vi "Help Seal.vi"(0 "Signals":T2, 5 "Pressure Controls":T1, 7 "Seal Parameters":refnum<vi>, 9 "Suction Parameters":refnum<vi>, 11 "error in (no error)":errorcluster, 13 "Dialog Indicator":refnum<vi>, 14 "Abort":refnum<vi>) -> (10 "Seal":bool, 15 "error out":errorcluster)   [LabVIEW 2012, in "Autopatcher Daemon.lvlib"]
uses:
  Autopatcher Daemon.lvlib
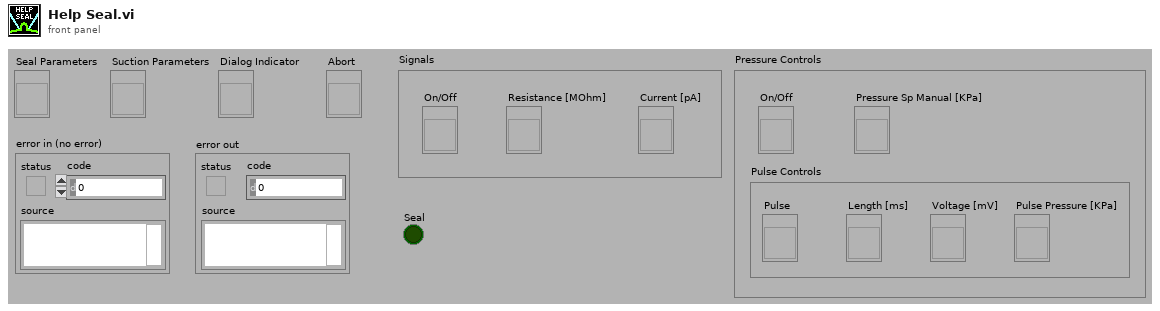
[diagram p1: front panel]
types:
  T1 = cluster{"On/Off":refnum<vi>, "Pulse Controls":cluster{"Pulse":refnum<vi>, "Length [ms]":refnum<vi>, "Voltage [mV]":refnum<vi>, "Pulse Pressure [KPa]":refnum<vi>}, "Pressure Sp Manual [KPa]":refnum<vi>}
  T2 = cluster{"On/Off":refnum<vi>, "Resistance [MOhm]":refnum<vi>, "Current [pA]":refnum<vi>}
  T3 = cluster{"Seal Target [MOhm]":dbl, "Stability Threhsold [%]":dbl, "Seal Timeout [s]":dbl, "Stability Refresh [ms]":dbl}
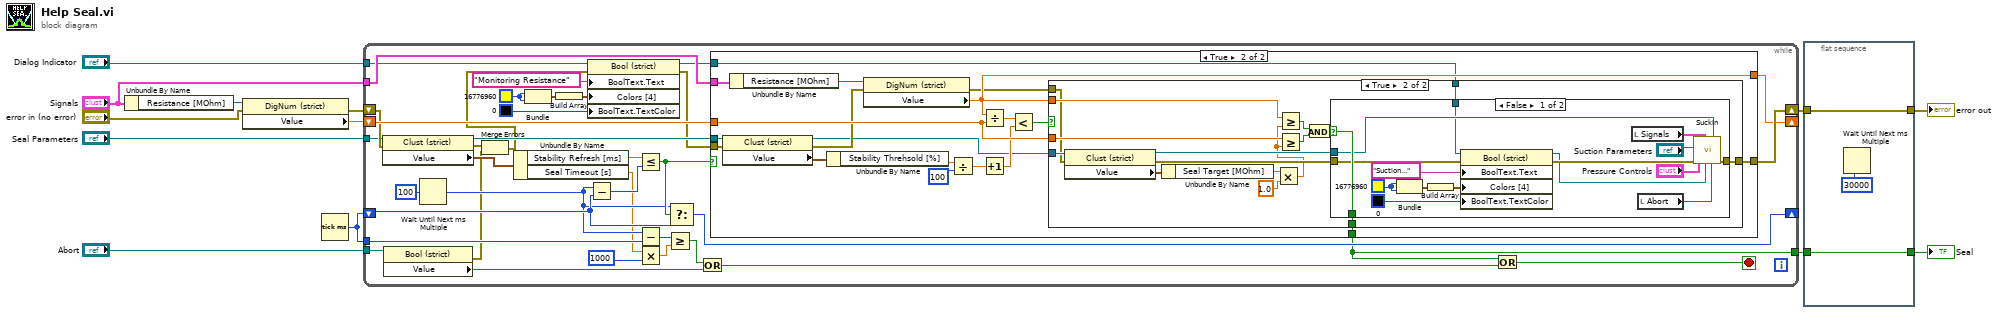
[diagram p0: block diagram]
diagram:
  n1 = Unbundle By Name("Signals") -> ("Resistance [MOhm]"=w12:refnum<vi>)
  n2 = property class="DigNum (strict)"(reference=w12, error in="error in (no error)") -> (error out=w10:errorcluster, "Value"=w11:dbl)  [unwired: 1 out]
  n3 = Tick Count (ms)() -> (millisecond timer value=w8:u32)
  n4 = while {
    shift-right: [w31] -> _
    shift-left: w8 -> [w50]
    tunnel: w8 -> [w47]
    shift-right: [w30] -> _
    shift-left: w11 -> [w45]
    tunnel: [w14] -> w13
    tunnel: "Abort" -> [w29]
    tunnel: "Signals" -> [w20]
    tunnel: "Seal Parameters" -> [w37]
    shift-right: [w43] -> w3
    shift-left: w10 -> [w38]
    tunnel: "Dialog Indicator" -> [w16]
    stop <- w44 stop-if-true
    w21 = u32 16776960
    n5 = property class="Clust (strict)"(reference=w37, error in=w38) -> (reference out=w36:refnum<vi>, error out=w27:errorcluster, "Value"=w35:T3)
    n6 = property class="Bool (strict)"(reference=w29) -> (error out=w26:errorcluster, "Value"=w33:bool)  [unwired: 1 in, 1 out]
    n7 = Wait Until Next ms Multiple(millisecond multiple=u32 100) -> (millisecond timer value=w39:u32)
    n8 = Merge Errors(w27, w26) -> (w18:errorcluster)
    n9 = Unbundle By Name(w35) -> ("Stability Refresh [ms]"=w15:dbl, "Seal Timeout [s]"=w28:dbl)
    n10 = Bundle(w21, w21) -> (w22:cluster{u32, u32})  [unwired: 1 in]
    n11 = Build Array(w22) -> (w23:cluster{u32, u32}[])
    n12 = property class="Bool (strict)"(reference=w16, error in=w18, "BoolText.Text"="Monitoring Resistance" ("Boolean Text.Text"), "Colors [4]"=w23, "BoolText.TextColor"=u32 0) -> (reference out=w17:refnum<vi>, error out=w19:errorcluster)
    n13 = Subtract(x=w39, y=w50) -> (x-y=w48:u32)
    n14 = Less Or Equal?(x=w15, y=w48) -> (x <= y?=w49:bool)
    n15 = Subtract(x=w39, y=w47) -> (x-y=w46:u32)
    n16 = Multiply(x=w28, y=u32 1000) -> (x*y=w40:dbl)
    n17 = Greater Or Equal?(x=w46, y=w40) -> (x >= y?=w34:bool)
    n18 = Select(t=w39, s=w49, f=w50) -> (s? t:f=w31:u32)
    n19 = Or(x=w34, y=w33) -> (x .or. y?=w41:bool)
    n20 = case shown="True" w49 {
      selector: w49 -> [w52 _]
      tunnel: w45 -> [w53 w70]
      tunnel: [w53 w67] -> w30
      tunnel: [w52 w69] -> w14
      tunnel: [w51 w68] -> w43
      tunnel: w20 -> [_ w55]
      tunnel: w36 -> [_ w60]
      tunnel: w19 -> [w51 w59]
      tunnel: w17 -> [_ w54]
      frame False {
      }
      frame True {
        n21 = property class="Clust (strict)"(reference=w60, error in=w59) -> (reference out=w57:refnum<vi>, error out=w58:errorcluster, "Value"=w62:T3)
        n22 = Unbundle By Name(w55) -> ("Resistance [MOhm]"=w61:refnum<vi>)
        n23 = Unbundle By Name(w62) -> ("Stability Threhsold [%]"=w66:dbl)
        n24 = property class="DigNum (strict)"(reference=w61, error in=w58) -> (error out=w56:errorcluster, "Value"=w67:dbl)  [unwired: 1 out]
        n25 = Divide(x=w66, y=u32 100) -> (x/y=w65:dbl)
        n26 = Divide(x=w67, y=w70) -> (x/y=w72:dbl)
        n27 = Increment(x=w65) -> (x+1=w63:dbl)
        n28 = Less?(x=w72, y=w63) -> (x < y?=w71:bool)
        n29 = case shown="True" w71 {
          selector: w71 -> [w74 _]
          tunnel: w67 -> [_ w87]
          tunnel: w70 -> [_ w86]
          tunnel: [w74 w85] -> w69
          tunnel: [w73 w84] -> w68
          tunnel: w57 -> [_ w82]
          tunnel: w56 -> [w73 w81]
          tunnel: w54 -> [_ w78]
          frame False {
          }
          frame True {
            n30 = property class="Clust (strict)"(reference=w82, error in=w81) -> (reference out=w80:refnum<vi>, error out=w79:errorcluster, "Value"=w83:T3)
            n31 = Unbundle By Name(w83) -> ("Seal Target [MOhm]"=w77:dbl)
            n32 = Multiply(x=w77, y=1.0) -> (x*y=w75:dbl)
            n33 = Greater Or Equal?(x=w87, y=w75) -> (x >= y?=w90:bool)
            n34 = Greater Or Equal?(x=w86, y=w75) -> (x >= y?=w89:bool)
            n35 = And(x=w90, y=w89) -> (x .and. y?=w88:bool)
            n36 = case shown="False" w88 {
              selector: w88 -> [w106 w108]
              tunnel: [w106 w108] -> w85
              tunnel: [w105 w107] -> w84
              tunnel: w80 -> [w101 _]
              tunnel: w79 -> [w98 w107]
              tunnel: w78 -> [w99 _]
              frame False {
                w96 = u32 16776960
                n37 = Bundle(w96, w96) -> (w95:cluster{u32, u32})  [unwired: 1 in]
                n38 = Build Array(w95) -> (w94:cluster{u32, u32}[])
                n39 = property class="Bool (strict)"(reference=w99, error in=w98, "BoolText.Text"="Suction..." ("Boolean Text.Text"), "Colors [4]"=w94, "BoolText.TextColor"=u32 0) -> (reference out=w91:refnum<vi>, error out=w100:errorcluster)
                n40 = local read "Signals"() -> (w104:T2)
                n41 = local read "Abort"() -> (w92:refnum<vi>)
                n42 = call "Suckin.vi"("Abort"=w92, "Dialog Indicator"=w91, "Signals"=w104, "error in (no error)"=w100, "Pressure Controls"="Pressure Controls", "Suction Parameters"="Suction Parameters", "Seal Parameters"=w101) -> ("error out"=w105:errorcluster)  [unwired: 3 in, 1 out]
              }
              frame True {
              }
            }
          }
        }
      }
    }
    n43 = Or(x=w14, y=w41) -> (x .or. y?=w44:bool)
  }
  n44 = flat-sequence {
    tunnel: w13 -> [w109]
    tunnel: w3 -> [w110]
    tunnel: [w110] -> w2
    tunnel: [w109] -> w1
    frame #0 {
      n45 = Wait Until Next ms Multiple(millisecond multiple=u32 30000) -> ()  [unwired: 1 out]
    }
  }
  "error out" <- w2
  "Seal" <- w1
